vi "string_to_main_trigger.vi"(8 "error in (no error)":errorcluster, 10 "trigger string":string) -> (0 "error out":errorcluster, 2 "main trigger":T1)   [LabVIEW 2017]
uses:
  type_definitions/enumerations/main_trigger_enum.ctl
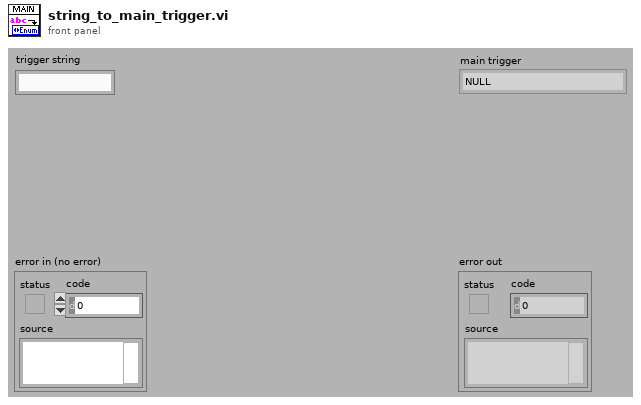
[diagram p1: front panel]
types:
  T1 = typedef "main_trigger_enum.ctl" = enum16{"NULL", "initialise", "terminate", "start", "stop", "change objective", "change experimentController", "change imagingMode", "save notebook", "started saving", "finished saving", "expCtr ready", "expCtr missing", "imgMd ready", "imgMd missing", "scanHd ready", "scanHd missing", "DAQ ready", "DAQ missing", "imgAsm ready", "imgAsm missing", "dataColl ready", "dataColl missing", "display ready", "display missing", "analysr ready", "analysr missing", "instrmnt ready", "instrmnt missing", "stimltr ready", "stimltr missing", "stage ready", "stage missing"}
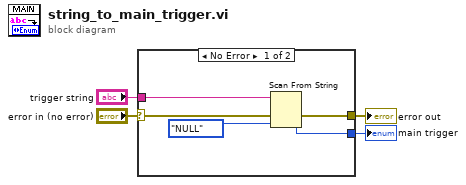
[diagram p0: block diagram]
diagram:
  n1 = case shown="No Error" "error in (no error)" {
    selector: "error in (no error)" -> [w9 w10]
    tunnel: [w8 w10] -> w3
    tunnel: "trigger string" -> [w7 _]
    tunnel: [w5 _] -> w1
    frame No Error {
      n2 = Scan From String(input string=w7, error in=w9, default 1=main_trigger_enum."NULL" ("trigger")) -> (error out=w8:errorcluster, output 1=w5:T1)  [unwired: 2 in, 2 out]
    }
    frame Error {
    }
  }
  "error out" <- w3
  "main trigger" <- w1
